vi "to_json.vi"(8 "error in":errorcluster, 11 "workspace in":refnum<class "workspace.lvclass">) -> (0 "error out":errorcluster, 2 "json":string, 3 "workspace out":refnum<class "workspace.lvclass">)   [LabVIEW 2020, in "nominal types.lvlib" / "workspace.lvclass"]
uses:
  workspace.lvclass
  workspace.lvclass/workspace.ctl
  bf7b01e1-8110-4372-be0e-405f04d60bdb.vi
  <vilib>/JDP Science/JSONtext/Variant to JSON Text.vi
  <vilib>/JDP Science/JSONtext/LVClass Serializer/JSONtext LVClass Serializer.lvclass
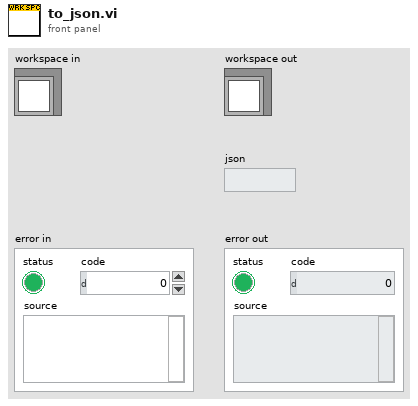
[diagram p1: front panel]
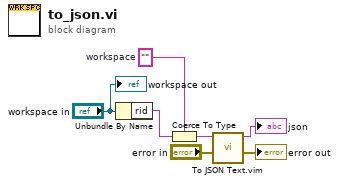
[diagram p0: block diagram]
diagram:
  w5 = ""  # workspace
  n1 = Unbundle By Name("workspace in") -> ("rid"=w6:string)
  n2 = Coerce To Type(0:w6, 1:w5) -> (2:w4:string)
  n3 = call "To JSON Text.vim"("error in (no error)"="error in", "Anything"=w4) -> ("error out"=→"error out":errorcluster, "<JSON>"=→"json":string)  [unwired: 8 in]
  "workspace out" <- "workspace in"
